vi "Release Session.vi"(0 "Session Handle":T1, 11 "error in (no error)":errorcluster, 13 "force destroy? (F)":bool) -> (15 "error out":errorcluster)   [LabVIEW 2014, in "Serial Session.lvclass"]
doc: "Closes the serial port once all sessions have been released."
uses:
  Serial Session.lvclass
  <userlib>/_Session Fwk/Session - Root.lvclass
  Typedefs/Session Handle.ctl
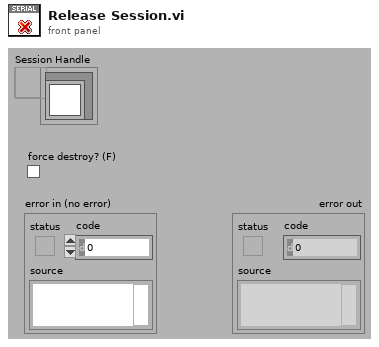
[diagram p1: front panel]
types:
  T1 = typedef "Serial Session.lvclass/Session Handle.ctl" = refnum<data-value>
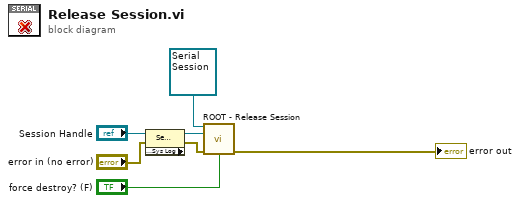
[diagram p0: block diagram]
diagram:
  n1 = property class="Serial Session" props=["Public:Accessors:Sys Log"](reference="Session Handle", error in="error in (no error)") -> (reference out=w3:T1, error out=w1:errorcluster)  [unwired: 1 out]
  n2 = call <userlib>:"ROOT - Release Session.vi"("OBJ - Session in"=refnum<class "Serial Session.lvclass"> refnum ("Session class"), "Session Handle in"=w3, "error in (no error)"=w1, "force destroy? (F)"="force destroy? (F)") -> ("error out"=→"error out":errorcluster)  [unwired: 10 in, 1 out]
